vi "Real Uncertain Min Finder.vi"(4 "data":variant, 5 "x":dbl) -> (2 "f(x)":dbl)   [LabVIEW 2011]
uses:
  BaesDataTypeDefinition.ctl
panel:
  in  "cluster":T2
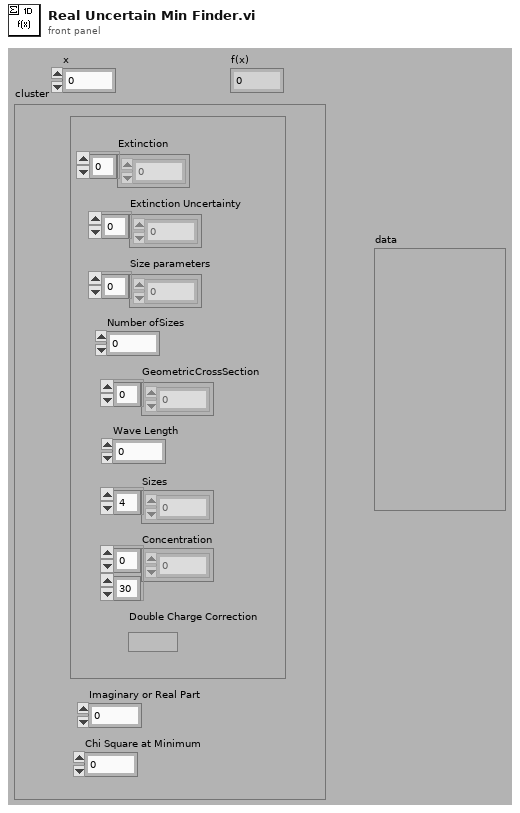
[diagram p1: front panel]
types:
  T1 = typedef "BaesDataTypeDefinition.ctl" = cluster{"Extinction":dbl[], "Extinction Uncertainty":dbl[], "Size parameters":dbl[], "Number ofSizes":dbl, "GeometricCrossSection":dbl[], "Wave Length":dbl, "Sizes":dbl[], "Concentration":dbl[][], "Double Charge Correction":bool}
  T2 = cluster{"Imaginary or Real Part":dbl, "Chi Square at Minimum":dbl, "Extinction ExtinctionUncertainity Size parameter and Number ofS sizes":T1}
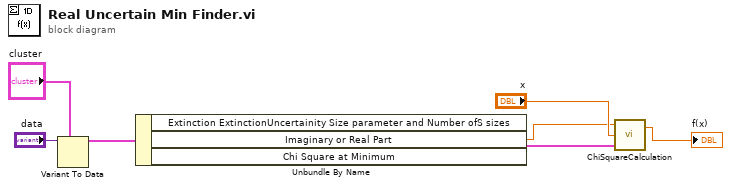
[diagram p0: block diagram]
diagram:
  n1 = Variant To Data(type="cluster", Variant="data") -> (data=w5:T2)  [unwired: 1 in, 1 out]
  n2 = Unbundle By Name(w5) -> ("Extinction ExtinctionUncertainity Size parameter and Number ofS sizes"=w7:T1, "Imaginary or Real Part"=w2:dbl)  [unwired: 1 out]
  n3 = call "ChiSquareCalculation.vi"("Extinction ExtinctionUncertainity Size parameter and Number ofS sizes 2"=w7, "refractive index, imaginary"="x", "refractive index, real"=w2) -> ("Chi Squared"=→"f(x)":dbl)  [unwired: 1 out]
